vi "Movimiento_Helicoidal.vi"() -> ()   [LabVIEW 2017]
uses:
  <vilib>/Motion/Express/_s/nimc.fb.arcMove.startArcMove.coordinate.modeHelical.0.vi
  <vilib>/Motion/BlockNode/FB.NIMotion.xnode
panel:
  in  "linear travel":dbl
  in  "travel angle":dbl=270.0
  in  "start angle":dbl
  in  "radius":dbl=1000.0
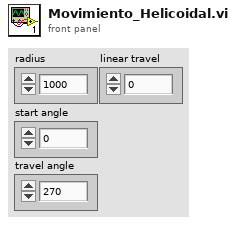
[diagram p1: front panel]
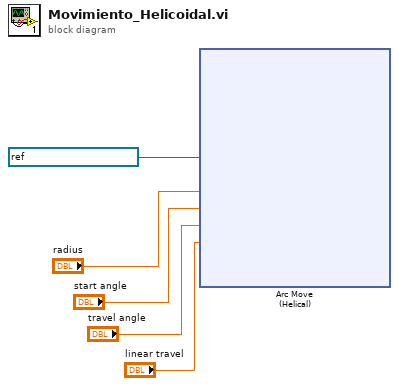
[diagram p0: block diagram]
diagram:
  n1 = xnode "Arc Move\n(Helical)"("resource"=refnum<k21> "Coordinate Space 1", "radius"="radius", "start angle"="start angle", "travel angle"="travel angle", "linear travel"="linear travel") -> ()  [unwired: 4 in, 3 out]
